vi "Add AO.vi"(8 "error in (no error)":errorcluster, 10 "Physical Channel Number":i32, 11 "Device Item Ref in":T1 format="%.0x") -> (0 "error out":errorcluster, 3 "Parent Ref out":T1 format="%.0x")   [LabVIEW 2020, in "Waveform Analog Output System Explorer.lvlib"]
doc: "Add an Analog Output channel based on the physical channel specified"
uses:
  Waveform Analog Output System Explorer.lvlib
  <vilib>/NI VeriStand/Custom Device API/Custom Device Item Ref.ctl
  <vilib>/NI VeriStand/Custom Device API/Custom Device Channel.ctl
  <vilib>/NI VeriStand/Custom Device API/Custom Device Channel Type.ctl
  Shared/Constants.vi
  <vilib>/NI VeriStand/Custom Device API/Custom Device API.lvlib
  Shared/Waveform Analog Output Shared.lvlib
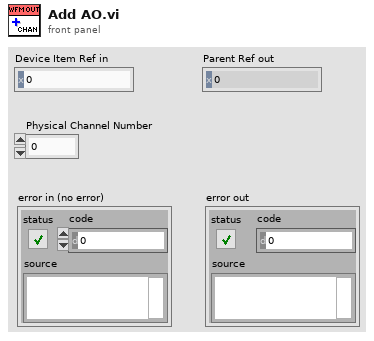
[diagram p1: front panel]
types:
  T1 = typedef "Custom Device API.lvlib/Custom Device Item Ref.ctl" = u64
  T2 = typedef "Custom Device API.lvlib/Custom Device Channel.ctl" = cluster{"Type":T3, "Units":string, "Default Value":dbl, "Faultable":bool, "Scalable":bool}
  T3 = typedef "Custom Device API.lvlib/Custom Device Channel Type.ctl" = enum16{"Input", "Output"}
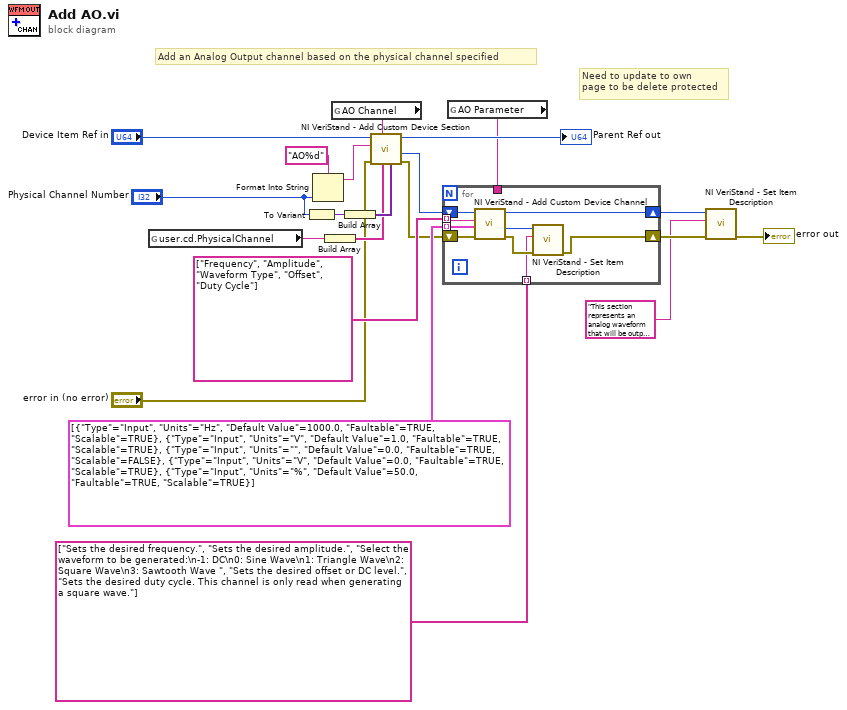
[diagram p0: block diagram]
diagram:
  # "Need to update to own\npage to be delete protected"
  # "Add an Analog Output channel based on the physical channel specified"
  n1 = global read "Constants.vi" "user.cd.PhysicalChannel"() -> (w12:string)
  n2 = To Variant(anything="Physical Channel Number") -> (Variant=w15:variant)
  n3 = Format Into String(format string="AO%d", "Physical Channel Number") -> (resulting string=w10:string)  [unwired: 2 in, 1 out]
  n4 = Build Array(w12) -> (w13:string[])
  n5 = global read "Constants.vi" "AO Channel"() -> (w8:string)
  n6 = Build Array(w15) -> (w16:variant[])
  n7 = call <vilib>:"NI VeriStand - Add Custom Device Section.vi"("Property Values"=w16, "Property names"=w13, "GUID (Default Section)"=w8, "error in (no error)"="error in (no error)", "Section Name"=w10, "Parent Ref in"="Device Item Ref in") -> ("error out"=w18:errorcluster, "Section Ptr"=w17:T1, "Parent Ref out"=→"Parent Ref out":T1)  [unwired: 2 in, 1 out]
  n8 = global read "Constants.vi" "AO Parameter"() -> (w6:string)
  n9 = for {
    shift-right: [w23] -> w3
    shift-left: w18 -> [w29]
    shift-right: [w28] -> w4
    shift-left: w17 -> [w30]
    tunnel: string[] ["Frequency", "Amplitude", "Waveform Type", "Offset", "Duty Cycle"] -> [w27] mode=indexing
    tunnel: T2[] [{"Type"=enum."Input", "Units"="Hz", "Default Value"=1000.0, "Faultable"=TRUE, "Scalable"=TRUE}, {"Type"=enum."Input", "Units"="V", "Default Value"=1.0, "Faultable"=TRUE, "Scalable"=TRUE}, {"Type"=enum."Input", "Units"="", "Default Value"=0.0, "Faultable"=TRUE, "Scalable"=FALSE}, {"Type"=enum."Input", "Units"="V", "Default Value"=0.0, "Faultable"=TRUE, "Scalable"=TRUE}, {"Type"=enum."Input", "Units"="%", "Default Value"=50.0, "Faultable"=TRUE, "Scalable"=TRUE}] -> [w26] mode=indexing
    tunnel: w6 -> [_]
    tunnel: string[] ["Sets the desired frequency.", "Sets the desired amplitude.", "Select the waveform to be generated:\n-1: DC\n0: Sine Wave\n1: Triangle Wave\n2: Square Wave\n3: Sawtooth Wave ", "Sets the desired offset or DC level.", "Sets the desired duty cycle. This channel is only read when generating a square wave."] -> [w22] mode=indexing
    n10 = call <vilib>:"NI VeriStand - Add Custom Device Channel.vi"("error in (no error)"=w29, "Channel"=w26, "Channel Name"=w27, "Parent Ref in"=w30) -> ("error out"=w24:errorcluster, "Channel Ref"=w25:T1, "Parent Ref out"=w28:T1)  [unwired: 4 in, 1 out]
    n11 = call <vilib>:"NI VeriStand - Set Item Description.vi"("error in (no error)"=w24, "Description"=w22, "Item Ref in"=w25) -> ("error out"=w23:errorcluster)  [unwired: 6 in, 2 out]
  }
  n12 = call <vilib>:"NI VeriStand - Set Item Description.vi"("error in (no error)"=w3, "Description"="This section represents an analog waveform that will be output on the physical channel listed above. You can manipulate this waveform by changing the VeriStand channels underneath this section.", "Item Ref in"=w4) -> ("error out"=→"error out":errorcluster)  [unwired: 6 in, 2 out]
